vi "TargetAndLoad2.vi"   [LabVIEW 2015]
uses:
  MotorPositionGlobals.vi
  GlobalVisionVars.vi
  VisionGlobals.vi
  GeneralGlobals.vi
types:
  T1 = typedef "WPI_DigitalOutputDevRef.ctl" = cluster{"DIO Channel":T2, "DevStatus":errorcluster}
  T2 = typedef "FPGA_DIOChannel.ctl" = enum8{"DIO 0", "DIO 1", "DIO 2", "DIO 3", "DIO 4", "DIO 5", "DIO 6", "DIO 7", "DIO 8", "DIO 9", "DIO MXP 0", "DIO MXP 1", "DIO MXP 2", "DIO MXP 3", "DIO MXP 4", "DIO MXP 5", "DIO MXP 6", "DIO MXP 7", "DIO MXP 8", "DIO MXP 9", "DIO MXP 10", "DIO MXP 11", "DIO MXP 12", "DIO MXP 13", "DIO MXP 14", "DIO MXP 15", "Invalid"}
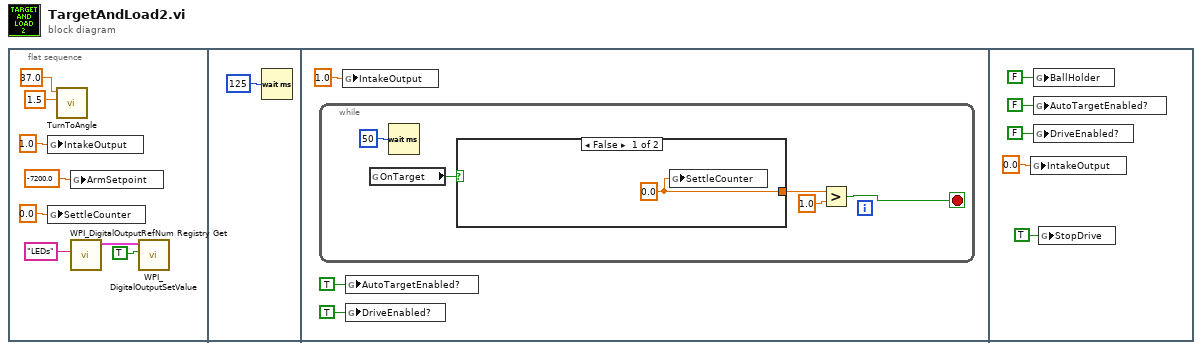
[diagram p0: block diagram]
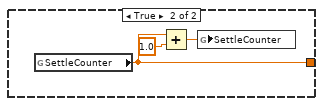
[diagram p2: hidden frame]
diagram:
  n1 = flat-sequence {
    frame #0 {
      n2 = global write "MotorPositionGlobals.vi" "IntakeOutput"(1.0 ("IntakeOutput")) -> ()
      n3 = global write "GlobalVisionVars.vi" "SettleCounter"(0.0 ("SettleCounter")) -> ()
      n4 = call "TurnToAngle.vi"("AllowedDeviation"=1.5, "GyroValue"=37.0) -> ()  [unwired: 10 in]
      n5 = global write "MotorPositionGlobals.vi" "ArmSetpoint"(-7200.0 ("ArmSetpoint")) -> ()
      n6 = call <vilib>:"WPI_DigitalOutputRefNum Registry Get.vi"("refnum name"="LEDs") -> ("DigitalOutputDevRef"=w4:T1)  [unwired: 9 in, 1 out]
      n7 = call <vilib>:"WPI_DigitalOutputSetValue.vi"("Value"=TRUE, "DigitalOutputDevRef"=w4) -> ()  [unwired: 8 in, 2 out]
    }
    frame #1 {
      n8 = Wait (ms)(milliseconds to wait=u32 125) -> ()  [unwired: 1 out]
    }
    frame #2 {
      n9 = while {
        stop <- w13 stop-if-true
        n10 = global read "GlobalVisionVars.vi" "OnTarget"() -> (w16:bool)
        n11 = Wait (ms)(milliseconds to wait=u32 50) -> ()  [unwired: 1 out]
        n12 = case shown="False" w16 {
          tunnel: [w18 w19] -> w14
          frame False {
            w18 = 0.0 ("SettleCounter")
            n13 = global write "GlobalVisionVars.vi" "SettleCounter"(w18) -> ()
          }
          frame True {
            n14 = global read "GlobalVisionVars.vi" "SettleCounter"() -> (w19:dbl)
            n15 = Add(x=w19, y=1.0) -> (x+y=w20:dbl)
            n16 = global write "GlobalVisionVars.vi" "SettleCounter"(w20) -> ()
          }
        }
        n17 = Greater?(x=w14, y=1.0) -> (0:w13:bool)
      }
      n18 = global write "MotorPositionGlobals.vi" "IntakeOutput"(1.0 ("IntakeOutput")) -> ()
      n19 = global write "VisionGlobals.vi" "AutoTargetEnabled?"(TRUE ("AutoTargetEnabled?")) -> ()
      n20 = global write "VisionGlobals.vi" "DriveEnabled?"(TRUE ("DriveEnabled?")) -> ()
    }
    frame #3 {
      n21 = global write "MotorPositionGlobals.vi" "IntakeOutput"(0.0 ("IntakeOutput")) -> ()
      n22 = global write "MotorPositionGlobals.vi" "BallHolder"(FALSE ("BallHolder")) -> ()
      n23 = global write "VisionGlobals.vi" "AutoTargetEnabled?"(FALSE ("AutoTargetEnabled?")) -> ()
      n24 = global write "VisionGlobals.vi" "DriveEnabled?"(FALSE ("DriveEnabled?")) -> ()
      n25 = global write "GeneralGlobals.vi" "StopDrive"(TRUE ("StopDrive")) -> ()
    }
  }
